vi "Write Command.vi"(8 "error in":errorcluster, 10 "command":string, 11 "GOLPI ref. in":T1={"pipe handle"={"lv_proc.dll file path"=path "", "process instance handle"=[]}, "fast read timeout [ms]"=500, "fast read settle time [ms]"=10, "fast read to multiple [ms]"=1, "max elements per input line"=100}) -> (0 "error out":errorcluster, 3 "GOLPI ref. out":T1={"pipe handle"={"lv_proc.dll file path"=path "", "process instance handle"=[]}, "fast read timeout [ms]"=500, "fast read settle time [ms]"=10, "fast read to multiple [ms]"=1, "max elements per input line"=100})   [LabVIEW 2013, in "GOLPI library.lvlib"]
doc: "Sends command to GNU Octave. End of line is added automatically if missing."
uses:
  GOLPI library.lvlib
  Private/Type Definitions/GOLPI reference Type Def.ctl
  LV Process.lvlibp/Pipe Handle.ctl
  LV Process.lvlibp
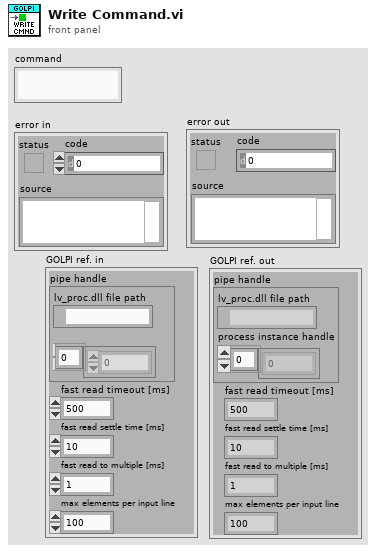
[diagram p1: front panel]
types:
  T1 = typedef "GOLPI library.lvlib/GOLPI reference Type Def.ctl" = cluster{"pipe handle":T2, "fast read timeout [ms]":u32, "fast read settle time [ms]":u32, "fast read to multiple [ms]":u32, "max elements per input line":u32}
  T2 = typedef "LV Process.lvlibp/Pipe Handle.ctl" = cluster{"lv_proc.dll file path":path, "process instance handle":u32[]}
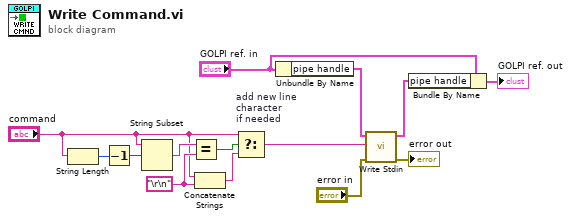
[diagram p0: block diagram]
diagram:
  w9 = "\r\n"
  n1 = String Length(string="command") -> (length=w13:i32)
  n2 = Decrement(x=w13) -> (x-1=w12:i32)
  n3 = String Subset(string="command", offset (0)=w12) -> (substring=w11:string)  [unwired: 1 in]
  n4 = Equal?(x=w11, y=w9) -> (x = y?=w10:bool)
  n5 = Concatenate Strings("command", w9) -> (w8:string)
  n6 = Select "add new line\ncharacter\nif needed"(t="command", s=w10, f=w8) -> (s? t:f=w6:string)
  n7 = Unbundle By Name("GOLPI ref. in") -> ("pipe handle"=w2:T2)
  n8 = call "Write Stdin.vi"("error in"="error in", "write buffer"=w6, "pipe in"=w2) -> ("error out"=→"error out":errorcluster, "pipe out"=w1:T2)  [unwired: 6 in, 1 out]
  n9 = Bundle By Name(cluster="GOLPI ref. in", "pipe handle"=w1) -> (→"GOLPI ref. out":T1)
